vi "Keithley 2400 - Init.vi"(8 "limite:":dbl=2e-06, 11 "Porta:":refnum<visa-resource-name>="COM5") -> ()   [LabVIEW 2018]
uses:
  <vilib>/Instr/_visa.llb/VISA Configure Serial Port (Instr).vi
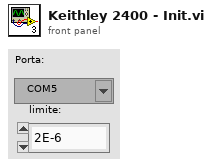
[diagram p1: front panel]
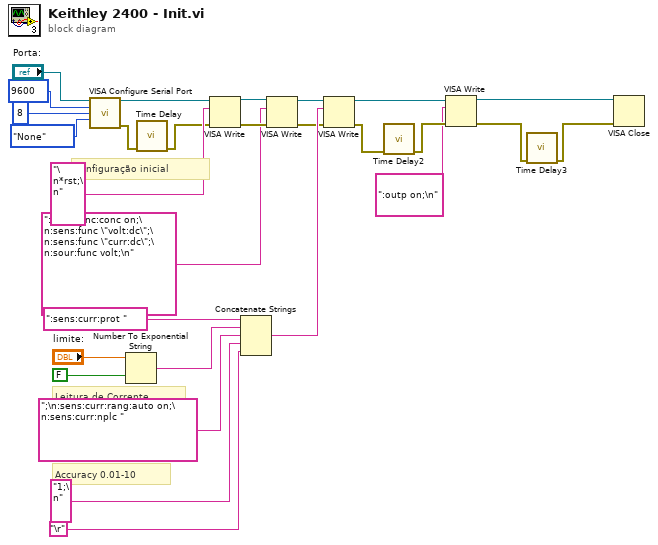
[diagram p0: block diagram]
diagram:
  # "Leitura de Corrente"
  # "Configuração inicial"
  # "Accuracy 0.01-10"
  n1 = call-poly "VISA Configure Serial Port"("VISA resource name"="Porta:", "baud rate (9600)"=u32 9600, "data bits (8)"=u16 8, "parity (0:none)"=enum16{"None", "Odd", "Even", "Mark", "Space"}."None") -> ("VISA resource name out"=w14:refnum<visa-resource-name>, "error out"=w13:errorcluster)  [unwired: 10 in]
  n2 = Number To Exponential String(number="limite:", 1:FALSE ("use system decimal point (T)")) -> (E-format string=w17:string)  [unwired: 2 in]
  n3 = call "Time Delay"("error in (no error)"=w13) -> ("error out"=w18:errorcluster)  [unwired: 10 in]
  n4 = VISA Write(VISA resource name=w14, write buffer="\n*rst;\n" ("string"), error in (no error)=w18) -> (VISA resource name out=w20:refnum<visa-resource-name>, error out=w28:errorcluster)  [unwired: 1 out]
  n5 = Concatenate Strings(":sens:curr:prot " ("string"), w17, ";\n:sens:curr:rang:auto on;\n:sens:curr:nplc " ("string"), "1;\n" ("string"), "\r") -> (w24:string)
  n6 = VISA Write(VISA resource name=w20, write buffer=":sens:func:conc on;\n:sens:func \"volt:dc\";\n:sens:func \"curr:dc\";\n:sour:func volt;\n" ("string"), error in (no error)=w28) -> (VISA resource name out=w25:refnum<visa-resource-name>, error out=w22:errorcluster)  [unwired: 1 out]
  n7 = VISA Write(VISA resource name=w25, write buffer=w24, error in (no error)=w22) -> (VISA resource name out=w21:refnum<visa-resource-name>, error out=w23:errorcluster)  [unwired: 1 out]
  n8 = call "Time Delay2"("error in (no error)"=w23) -> ("error out"=w19:errorcluster)  [unwired: 10 in]
  n9 = VISA Write(VISA resource name=w21, write buffer=":outp on;\n", error in (no error)=w19) -> (VISA resource name out=w6:refnum<visa-resource-name>, error out=w2:errorcluster)  [unwired: 1 out]
  n10 = call "Time Delay3"("error in (no error)"=w2) -> ("error out"=w1:errorcluster)  [unwired: 10 in]
  n11 = VISA Close(VISA resource name=w6, error in (no error)=w1) -> ()  [unwired: 1 out]
